vi "Static Read.vi"(8 "error in (no error)":errorcluster, 11 "Abs_Variant in":refnum<class "Abs_Variant.lvclass">) -> (0 "error out":errorcluster, 2 "Variant":variant, 3 "Abs_Variant out":refnum<class "Abs_Variant.lvclass">)   [LabVIEW 2021, in "Abs_Variant.lvclass"]
uses:
  Abs_Variant.lvclass
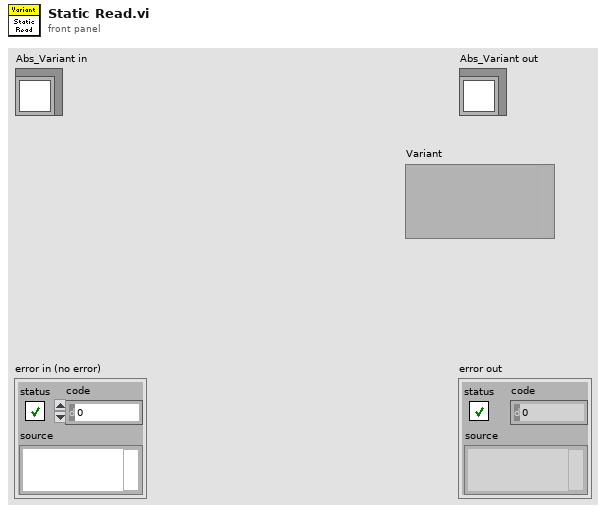
[diagram p1: front panel]
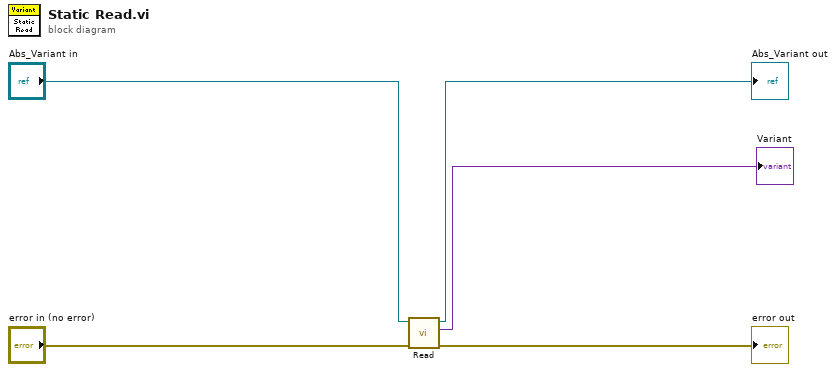
[diagram p0: block diagram]
diagram:
  n1 = call-dynamic "Read.vi"("error in (no error)"="error in (no error)", "Abs_Variant in"="Abs_Variant in") -> ("error out"=→"error out":errorcluster, "Variant"=→"Variant":variant, "Abs_Variant out"=→"Abs_Variant out":refnum<class "Abs_Variant.lvclass">)  [unwired: 7 in]
